vi "SV Stationary Loudness (Octave_2014) (1 Ch).vi"(0 "octave spectrum":T5={"nominal frequencies [Hz]"=[25.0, 31.5, 40.0, 50.0, 63.0, 80.0, 100.0, 125.0, 160.0, 200.0, 250.0, 315.0, 400.0, 500.0, 630.0, 800.0, 1000.0, 1250.0, 1600.0, 2000.0, 2500.0, 3150.0, 4000.0, 5000.0, 6300.0, 8000.0, 10000.0, 12500.0], "band power"=[-99.0, -99.0, -99.0, -99.0, -99.0, -99.0, -99.0, -99.0, -99.0, -99.0, -99.0, -99.0, -99.0, -99.0, 20.0, 40.0, 60.0, 40.0, 20.0, -99.0, -99.0, -99.0, -99.0, -99.0, -99.0, -99.0, -99.0, -99.0]} {"band power" format="%.2f"; "nominal frequencies [Hz]" format="%.2f"}, 1 "diffuse field":bool, 9 "octave info":T1={"standard"=enum."IEC 61260", "bandwidth"=enum."1/3 octave", "low band"=-16, "high band"=11, "weighting filter"=0, "dB reference"=2e-05, "dB On"=TRUE, "unit label"="Pa^2 rms|SV Units|dB ref 20u Pa", "channel name"="", "description"="", "engineering units"=2, "custom label"="", "spectrum type"=enum."power", "spectral density"=FALSE, "filters settled"=FALSE} {"engineering units" items=["custom..."=0, "V"=1, "A"=21, "C"=30, "pC"=31, "s"=32, "-"=29, "Pa"=2, "N"=20, "g"=3, "m/s^2"=4, "m/s"=5, "m"=6, "mm/s"=12, "mm"=13, "micron/s"=14, "micron"=15, "in/s^2"=7, "in/s"=8, "in"=9, "mil/s"=10, "mil"=11, "rad/s^2"=16, "rad/s"=17, "rad"=18, "deg/s^2"=26, "deg/s"=27, "deg"=28, "RPM"=22, "cycle/s^2"=23, "Hz"=24, "cycle"=25, "strain"=19]; "dB reference" format="%.2e"; "weighting filter" items=["Linear", "A-weighting", "B-weighting", "C-weighting", "ITU-R 468-4", "Dolby", "CCITT", "C-message", "Wb", "Wc", "Wd", "We", "Wf", "Wh", "Wj", "Wk", "Wm", "AES17 20 kHz lowpass", "AES17 40 kHz lowpass", "AES17 20 kHz highpass", "AES17 40 kHz highpass"]}, 11 "error in (no error)":errorcluster) -> (4 "specific loudness":cluster{dbl[], "Nm":dbl[]}(graph), 6 "loudness [Sone]":dbl format="%.2f", 8 "loudness level [Phon]":dbl format="%.2f", 10 "loudness info":T6, 15 "error out":errorcluster)   [LabVIEW 2017, in "SoundVib_SoundQuality.lvlib"]
doc: "Computes stationary loudness from the sound pressure signal waveform or the 1/3-octave band spectrum calculated over the frequency range 25 Hz to 12.5 kHz. Wire data to the <B>sound pressure signal [Pa]</B> input to determine the polymorphic instance to use or manually select the instance."
uses:
  <vilib>/addons/Sound and Vibration/svt_Sound Quality/SoundVib_SoundQuality.lvlib
  <vilib>/addons/_NISVFA/_Shared subVIs/Controls/svc_SQ Info.ctl
  <vilib>/addons/_NISVFA/_Shared subVIs/Controls/svc_Octave Info.ctl
  <vilib>/addons/_NISVFA/_Shared subVIs/Controls/svc_Octave Standard.ctl
  <vilib>/addons/_NISVFA/_Shared subVIs/Controls/svc_Weighting Filter Text Ring.ctl
  <vilib>/addons/_NISVFA/_Shared subVIs/Controls/svc_Engineering Units Text Ring.ctl
  <vilib>/addons/Sound and Vibration/svt_Octave_2014 standard/SVT Octave Spectrum Conversion (1 Ch).vi
  <vilib>/addons/Sound and Vibration/svt_Octave/SoundVib_Octave_2014 standard.lvlib
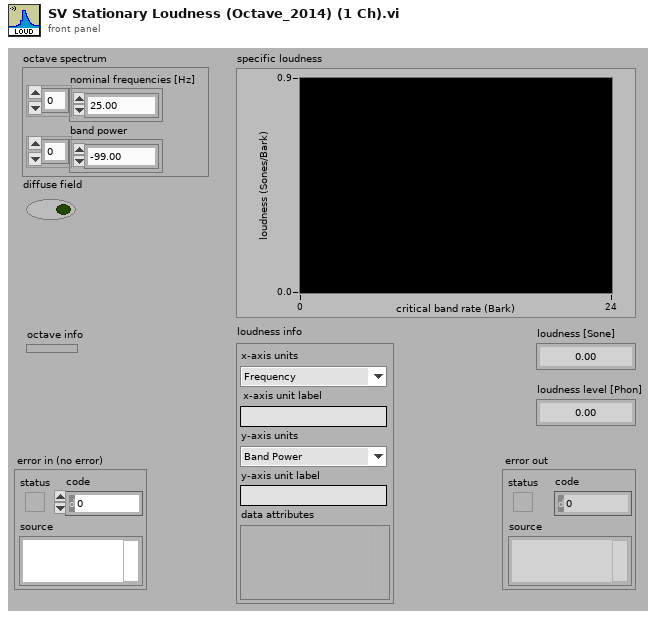
[diagram p1: front panel]
types:
  T1 = typedef "svc_Octave Info.ctl" = cluster{"standard":T2, "bandwidth":enum16{"1 octave", "1/3 octave", "1/6 octave", "1/12 octave", "1/24 octave"}, "low band":i32, "high band":i32, "weighting filter":T3, "dB reference":dbl, "dB On":bool, "unit label":string, "channel name":string, "description":string, "engineering units":T4, "custom label":string, "spectrum type":enum16{"power", "magnitude"}, "spectral density":bool, "filters settled":bool}
  T2 = typedef "svc_Octave Standard.ctl" = enum16{"ANSI S1.11", "IEC 61260"}
  T3 = typedef "svc_Weighting Filter Text Ring.ctl" = u16
  T4 = typedef "svc_Engineering Units Text Ring.ctl" = u16
  T5 = cluster{"nominal frequencies [Hz]":dbl[], "band power":dbl[]}
  T6 = typedef "svc_SQ Info.ctl" = cluster{"x-axis units":enum16{"Frequency", "Critical Band", "Critical Band Rate"}, "x-axis unit label":string, "y-axis units":enum16{"Band Power", "Level", "Loudness", "Sharpness", "Roughness", "Fluctuation Strength", "Tonality"}, "y-axis unit label":string, "data attributes":variant}
  T7 = enum16{"1 octave", "1/3 octave", "1/6 octave", "1/12 octave", "1/24 octave"}
  T8 = cluster{"linear/dB":enum16{"no change", "linear", "dB"}, "dB reference (0: no change)":dbl, "power/magnitude":enum16{"no change", "power", "magnitude"}, "spectral density":enum16{"no change", "spectrum", "spectral density"}}
  T9 = enum16{"Linear", "Linear + Bark edges", "Critical-band rates", "Critical band centers"}
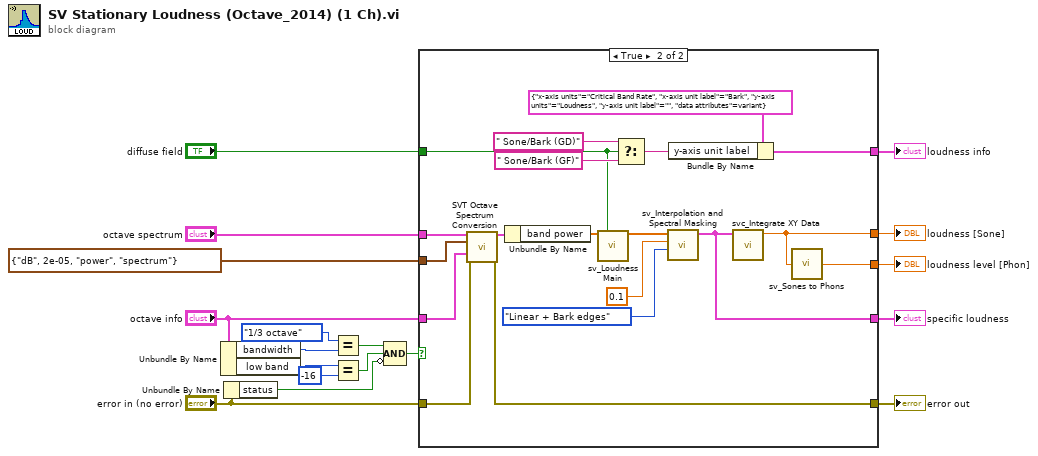
[diagram p0: block diagram]
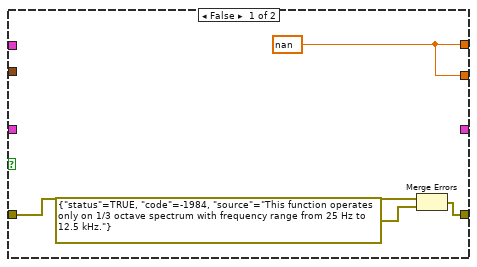
[diagram p2: hidden frame]
diagram:
  n1 = Unbundle By Name("octave info") -> ("bandwidth"=w9:T7, "low band"=w7:i32)
  n2 = Unbundle By Name("error in (no error)") -> ("status"=w3:bool)
  n3 = Equal?(x=T7."1/3 octave", y=w9) -> (x = y?=w5:bool)
  n4 = Equal?(x=w7, y=-16) -> (x = y?=w4:bool)
  n5 = Compound Arithmetic op=AND(w5, w4, invert w3) -> (w1:bool)
  n6 = case shown="True" w1 {
    tunnel: "diffuse field" -> [_ w39]
    tunnel: [w22 w38] -> w17
    tunnel: [w22 w36] -> w16
    tunnel: [_ w35] -> w15
    tunnel: [_ w32] -> w14
    tunnel: T8 {"linear/dB"=enum."dB", "dB reference (0: no change)"=2e-05, "power/magnitude"=enum."power", "spectral density"=enum."spectrum"} ("desired scaling") -> [_ w28]
    tunnel: "octave spectrum" -> [_ w27]
    tunnel: "error in (no error)" -> [w21 w25]
    tunnel: [w20 w24] -> w11
    tunnel: "octave info" -> [_ w23]
    frame False {
      w22 = nan ("integral(ydx)")
      n7 = Merge Errors(w21, errorcluster {"status"=TRUE, "code"=-1984, "source"="This function operates only on 1/3 octave spectrum with frequency range from 25 Hz to 12.5 kHz."} ("error in 2 (no error)")) -> (w20:errorcluster)
    }
    frame True {
      n8 = call-poly <vilib>:"SVT Octave Spectrum Conversion.vi"("octave spectrum"=w27, "desired scaling"=w28, "octave info in"=w23, "error in (no error)"=w25) -> ("converted octave spectrum"=w26:T5, "error out"=w24:errorcluster)  [unwired: 8 in, 2 out]
      n9 = Unbundle By Name(w26) -> ("band power"=w37:dbl[])
      n10 = call <vilib>:"sv_Loudness Main.vi"("1/3 OB Spectrum"=w37, "Diffuse Field?"=w39) -> ("Main Loudness"=w31:dbl[])  [unwired: 13 in]
      n11 = Select(t=" Sone/Bark (GD)", s=w39, f=" Sone/Bark (GF)") -> (s? t:f=w33:string)
      n12 = call <vilib>:"sv_Interpolation and Spectral Masking.vi"("interpolation type"=T9."Linear + Bark edges", "resolution (Bark)"=0.1, "Nm"=w31) -> ("specifc loudness"=w35:cluster{"Bark (X)":dbl[], "Nm (Y)":dbl[]})  [unwired: 8 in]
      n13 = Bundle By Name(cluster=T6 {"x-axis units"=enum."Critical Band Rate", "x-axis unit label"="Bark", "y-axis units"=enum."Loudness", "y-axis unit label"="", "data attributes"=variant} ("loudness info"), "y-axis unit label"=w33) -> (w32:T6)
      n14 = call <vilib>:"svc_Integrate XY Data.vi"("XY"=w35) -> ("integral(ydx)"=w36:dbl)  [unwired: 10 in]
      n15 = call <vilib>:"sv_Sones to Phons.vi"("Sones"=w36) -> ("Phons"=w38:dbl)  [unwired: 4 in]
    }
  }
  "loudness [Sone]" <- w16
  "loudness info" <- w14
  "loudness level [Phon]" <- w17
  "error out" <- w11
  "specific loudness" <- w15
